vi "WPI_SimpleGyro_Loop.vi"(8 "error in":errorcluster, 11 "SimpleGyroDevRef":T1) -> (0 "error out":errorcluster)   [LabVIEW 2015, in "SimpleGyro.lvlib"]
doc: "Periodically reads the SimpleGyro and makes data available to your robot project. Place this block within PeriodicTasks.vi."
uses:
  SimpleGyro.lvlib
  WPI_SimpleGyroDevRef.ctl
  <vilib>/Rock Robotics/SystemInterfaces/spilib/spi_bus.ctl
  <vilib>/Rock Robotics/WPI/SPI/WPI_SPIDevRef.ctl
  <vilib>/Platform/TimedLoop/XDataNode/timing_clust.ctl
  <vilib>/Platform/TimedLoop/XDataNode/nitl_modes.ctl
  <vilib>/Platform/TimedLoop/XDataNode/wakeup.ctl
  <vilib>/platform/TimedLoop/XDataNode/XDataNode.xnode
  <vilib>/Platform/TimedLoop/XDataNode/XDNodeRunTimeDep.lvlib
  <vilib>/ptbypt/NI_PtbyPt.lvlib
panel:
  out "Rate":dbl
  out "Device Found":bool
  out "Offset":dbl
  out "mean 2":dbl format="%0.2f"
  out "Angle":dbl
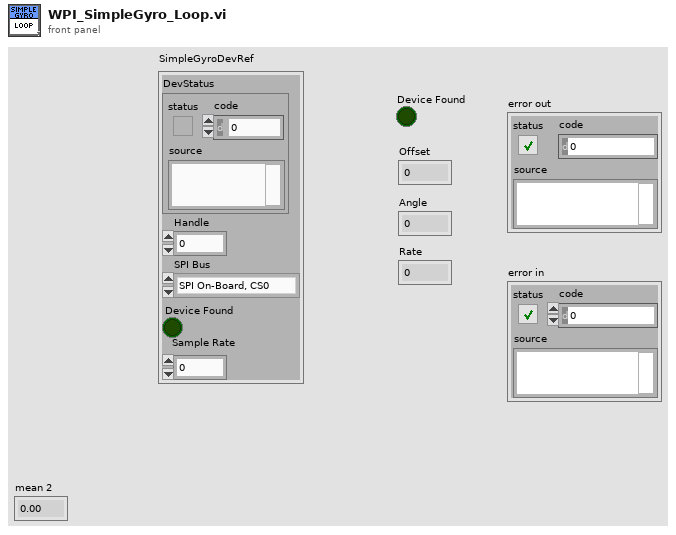
[diagram p1: front panel]
types:
  T1 = typedef "SimpleGyro.lvlib/WPI_SimpleGyroDevRef.ctl" = cluster{"DevStatus":errorcluster, "Handle":i32, "SPI Bus":T2, "Device Found":bool, "Sample Rate":dbl}
  T2 = typedef "spi_bus.ctl" = enum16{"SPI On-Board, CS0", "SPI On-Board, CS1", "SPI On-Board, CS2", "SPI On-Board, CS3", "SPI MXP", "Invalid"}
  T3 = typedef "WPI_SPIDevRef.ctl" = cluster{"DevStatus":errorcluster, "Handle":i32, "SPI Bus":T2}
  T4 = typedef "XDNodeRunTimeDep.lvlib/timing_clust.ctl" = cluster{"Expected End [f-1]":u64, "Actual End [f-1]":u64, "Finished Late? [f-1]":bool, "Expected End [i-1]":u64, "Actual End [i-1]":u64, "Finished Late? [i-1]":bool, "Expected Start [i]":u64, "Actual Start [i]":u64, "Expected Start [f]":u64, "Actual Start [f]":u64, "Source Name":string, "Structure Name":string, "Period":i64, "Deadline":i64, "Offset":i64, "Start":i64, "Priority":i32, "Timeout":i32, "Mode":T5, "Wakeup Reason":T6, "Error":errorcluster, "Source Type":string, "Secondary Source Type":string, "Global End Time":u64, "Global Start Time":u64, "Frame Duration":u64, "Iteration Duration":u64, "Assigned CPU":i32, "I/O Scan Engine Mode":u32}
  T5 = typedef "XDNodeRunTimeDep.lvlib/nitl_modes.ctl" = enum32{"No Change", "Process missed periods, maintain original phase", "Discard missed periods, maintain original phase", "Process missed periods, ignore original phase", "Discard missed periods, ignore original phase"}
  T6 = typedef "XDNodeRunTimeDep.lvlib/wakeup.ctl" = enum32{"Normal", "Aborted", "Asynchronous wakeup", "Timing source error", "Timed loop error", "Timeout"}
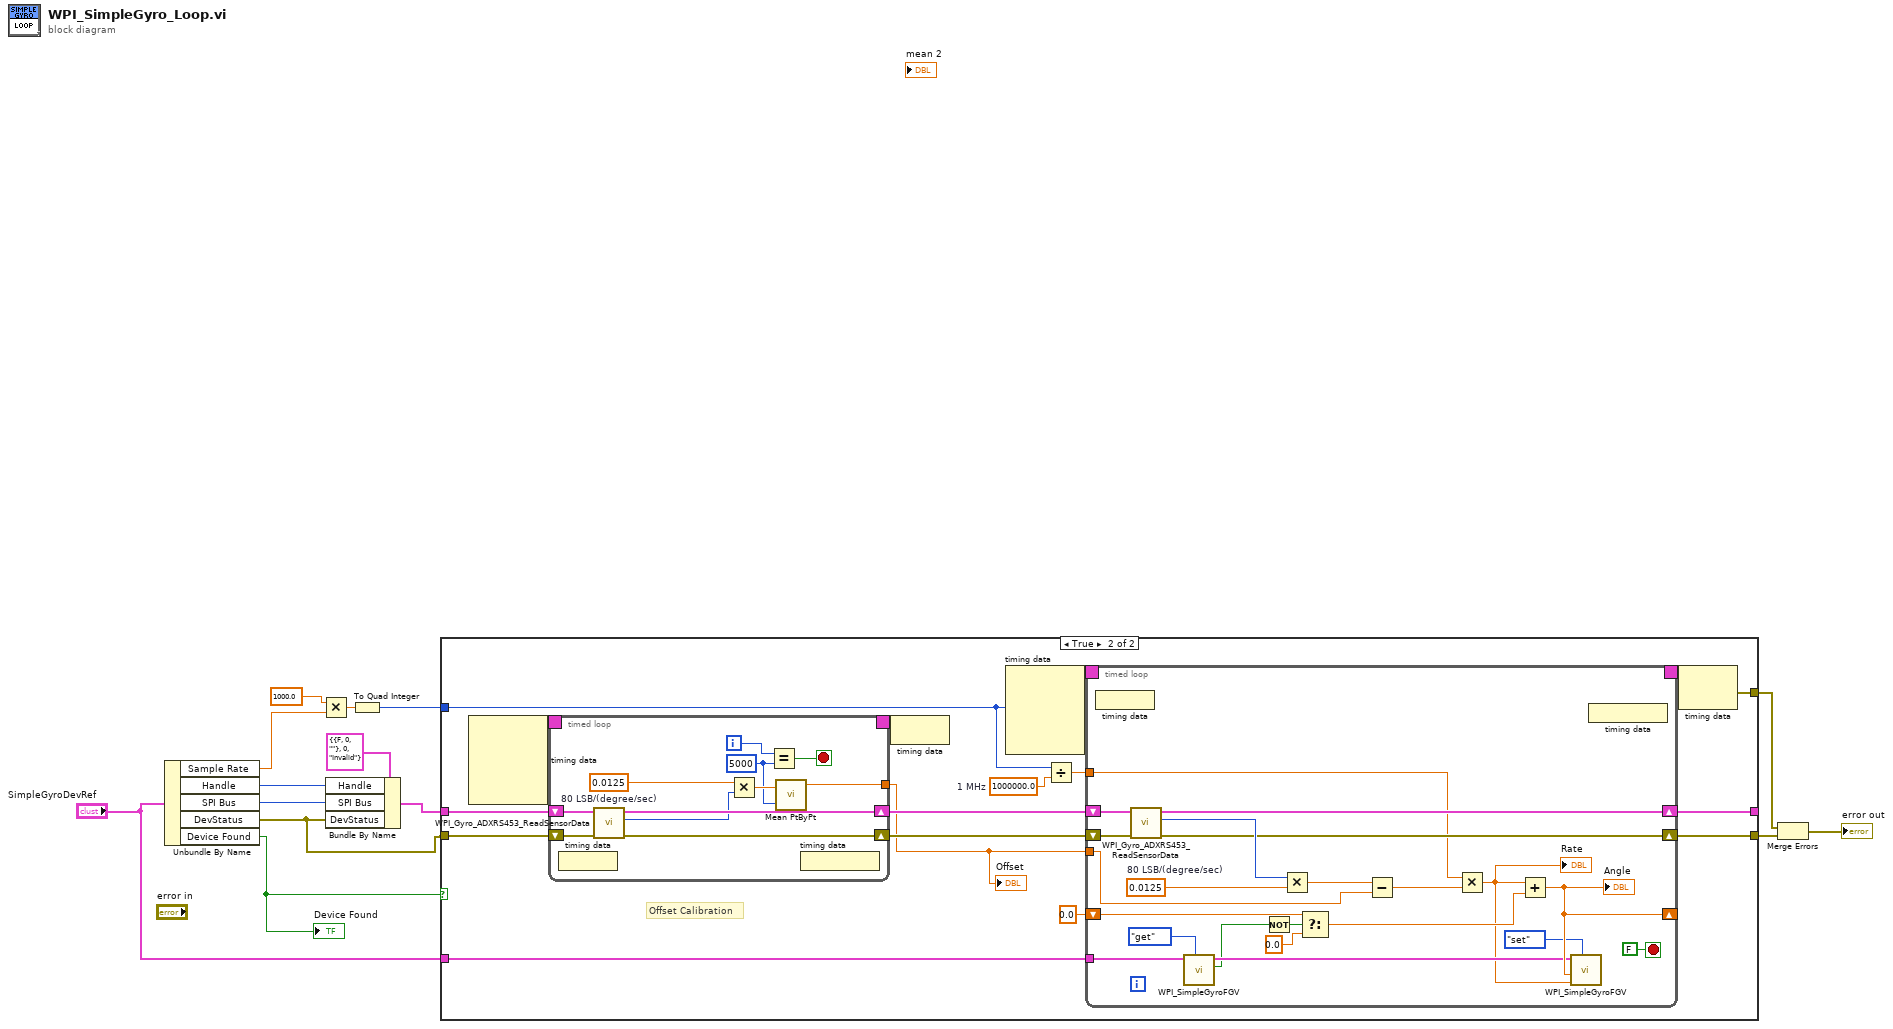
[diagram p0: block diagram]
diagram:
  n1 = Unbundle By Name("SimpleGyroDevRef") -> ("Sample Rate"=w4:dbl, "Handle"=w13:i32, "SPI Bus"=w12:T2, "DevStatus"=w1:errorcluster, "Device Found"=w11:bool)
  "Device Found" <- w11
  n2 = Multiply(x=1000.0 ("y"), y=w4) -> (x*y=w10:dbl)
  n3 = Bundle By Name(cluster=T3 {"DevStatus"={"status"=FALSE, "code"=0, "source"=""}, "Handle"=0, "SPI Bus"=enum."Invalid"} ("SPIDevRef out"), "Handle"=w13, "SPI Bus"=w12, "DevStatus"=w1) -> (w2:T3)
  n4 = To Quad Integer(1:w10) -> (0:w9:i64)
  n5 = case shown="True" w11 {
    tunnel: w2 -> [w16 w21]
    tunnel: w1 -> [w15 w20]
    tunnel: [w15 w31] -> w7
    tunnel: [w16 w30] -> _
    tunnel: w9 -> [_ w28]
    tunnel: "SimpleGyroDevRef" -> [_ w27]
    tunnel: [_ w26] -> w6
    frame False {
    }
    frame True {
      w24 = 1000000.0  # 1 MHz
      # "Offset Calibration"
      n6 = node-c288() -> (w23:T4)  [unwired: 4 in]
      n7 = timed-loop {
        shift-right: [w42] -> w19
        shift-left: w21 -> [w44]
        shift-right: [w39] -> w18
        shift-left: w20 -> [w43]
        timing: w23 -> [_]
        timing-out: [_] -> w22
        tunnel: [w37] -> w17
        i -> [w36]
        stop <- w35 stop-if-true
        w34 = 5000 ("y")
        w40 = 0.0125  # 80 LSB/(degree/sec)
        n8 = node-c288() -> ()  [unwired: 1 in]
        n9 = call "WPI_Gyro_ADXRS453_ReadSensorData.vi"("error in (no error)"=w43, "SPIDevRef in"=w44) -> ("error out"=w39:errorcluster, "Sensor Data (n-1)"=w41:i16, "SPIDevRef out"=w42:T3)  [unwired: 5 in, 2 out]
        n10 = Multiply(x=w40, y=w41) -> (x*y=w38:dbl)
        n11 = Equal?(x=w36, y=w34) -> (x = y?=w35:bool)
        n12 = call <vilib>:"Mean PtByPt.vi"("x"=w38, "sample length"=w34) -> ("mean"=w37:dbl)  [unwired: 2 in, 1 out]
        n13 = node-c288() -> ()  [unwired: 1 out]
      }
      "Offset" <- w17
      n14 = node-c288(w22) -> ()
      n15 = node-c288(w28) -> (w33:T4)  [unwired: 3 in]
      n16 = Divide(x=w28, y=w24) -> (x/y=w29:dbl)
      n17 = timed-loop {
        shift-right: [w68] -> w30
        shift-left: w19 -> [w70]
        shift-right: [w64] -> w31
        shift-left: w18 -> [w69]
        timing: w33 -> [_]
        timing-out: [_] -> w32
        shift-right: [w57] -> _
        shift-left: 0.0 -> [w65]
        tunnel: w29 -> [w53]
        tunnel: w27 -> [w59]
        tunnel: w17 -> [w51]
        stop <- FALSE stop-if-true
        w66 = 0.0125  # 80 LSB/(degree/sec)
        n18 = node-c288() -> ()  [unwired: 1 in]
        n19 = call "WPI_Gyro_ADXRS453_ReadSensorData.vi"("error in (no error)"=w69, "SPIDevRef in"=w70) -> ("error out"=w64:errorcluster, "Sensor Data (n-1)"=w67:i16, "SPIDevRef out"=w68:T3)  [unwired: 5 in, 2 out]
        n20 = call "WPI_SimpleGyroFGV.vi"("Operation"=enum16{"set", "get"}."get", "SimpleGyroDevRef"=w59) -> ("Reset?"=w54:bool, "SimpleGyroDevRef"=w55:T1)  [unwired: 6 in, 2 out]
        n21 = Not(x=w54) -> (.not. x?=w60:bool)
        n22 = Multiply(x=w67, y=w66) -> (x*y=w52:dbl)
        n23 = Select(t=w65, s=w60, f=0.0 ("t")) -> (s? t:f=w62:dbl)
        n24 = Subtract(x=w52, y=w51) -> (x-y=w50:dbl)
        n25 = Multiply(x=w53, y=w50) -> (x*y=w49:dbl)
        "Rate" <- w49
        n26 = Add(x=w49, y=w62) -> (x+y=w57:dbl)
        "Angle" <- w57
        n27 = call "WPI_SimpleGyroFGV.vi"("Operation"=enum16{"set", "get"}."set", "Rate"=w49, "Angle"=w57, "SimpleGyroDevRef"=w55) -> ()  [unwired: 4 in, 4 out]
        n28 = node-c288() -> ()  [unwired: 1 out]
      }
      n29 = node-c288(w32) -> (w26:errorcluster)
    }
  }
  n30 = Merge Errors(w6, w7) -> (→"error out":errorcluster)
